vi "PAGmem_test.vi"(8 "error in (no error)":errorcluster, 11 "PAQ-memory in":refnum<class "PAQ-memory.lvclass">) -> (0 "error out":errorcluster, 1 "TimeArray":dbl[](array[numeric]), 2 "PAQmemory":T1, 3 "PAQ-memory out":refnum<class "PAQ-memory.lvclass">)   [LabVIEW 2020, in "Sgraph_lib_V1.lvlib" / "PAQ-memory.lvclass"]
uses:
  PAQ-memory.lvclass
  controls/typedef_PAQdata.ctl
  PAQ-memory.lvclass/PAQ-memory.ctl
  FAMM.lvclass
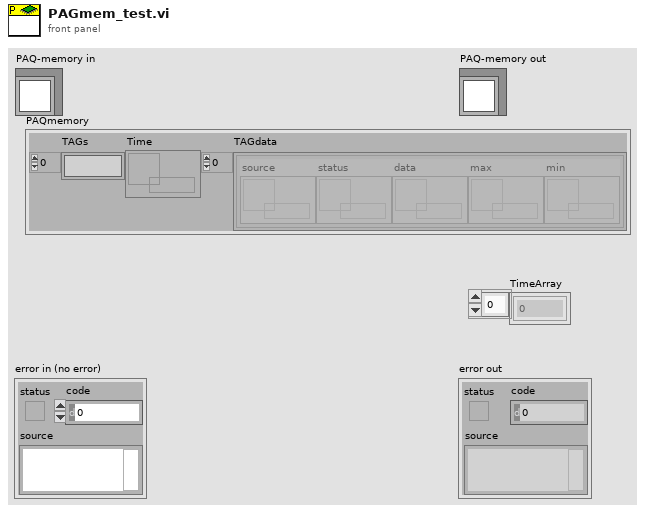
[diagram p1: front panel]
types:
  T1 = typedef "Sgraph_lib_V1.lvlib/FAMM.lvclass/typedef_PAQdata.ctl" = cluster{"TAGs":string[], "Time":refnum<data-value>, "TAGdata":cluster{"source":refnum<data-value>, "status":refnum<data-value>, "data":refnum<data-value>, "max":refnum<data-value>, "min":refnum<data-value>}[]}
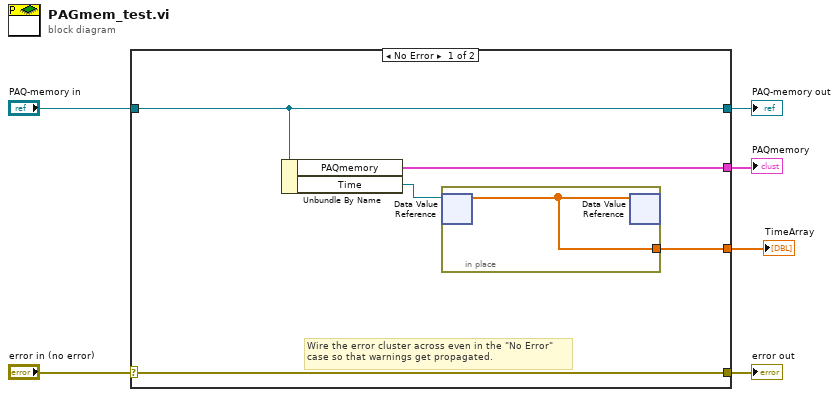
[diagram p0: block diagram]
diagram:
  n1 = case shown="No Error" "error in (no error)" {
    selector: "error in (no error)" -> [w11 w14]
    tunnel: [w11 w14] -> w5
    tunnel: [w10 w13] -> w3
    tunnel: "PAQ-memory in" -> [w10 w13]
    tunnel: [w9 _] -> w2
    tunnel: [w7 _] -> w1
    frame No Error {
      # "Wire the error cluster across even in the \"No Error\"\ncase so that warnings get propagated."
      n2 = Unbundle By Name(w10) -> ("PAQmemory"=w9:T1, "Time"=w8:refnum<data-value>)
      n3 = in-place {
        in-place-border: [w12] -> w7
        n4 = in-place-dvr #1(w8) -> (w12:dbl[])  [unwired: 1 out]
        n5 = in-place-dvr #1(w12) -> ()  [unwired: 2 out]
      }
    }
    frame Error {
    }
  }
  "error out" <- w5
  "PAQ-memory out" <- w3
  "PAQmemory" <- w2
  "TimeArray" <- w1
